vi "pll.vi"() -> ()   [LabVIEW 2020]
uses:
  <vilib>/Analysis/2dsp.llb/Real FFT.vi
  <vilib>/Analysis/baseanly.llb/Mean (DBL).vi
  <vilib>/Analysis/NI_AALBase.lvlib
  <vilib>/Analysis/NI_AALPro.lvlib
panel:
  out "Phase":dbl
  out "Input and Output Spectrum":waveform(dbl)[](graph)
  in  "milliseconds to wait":u32
  in  "iteration count":i32
  out "Input and Output vs Time":waveform(dbl)[](graph)
  in  "Loop Gain":dbl
  in  "Filter Length":i32=128
  in  "FFT size":i32=-1
  out "Frequency Estimate (Hz)":dbl
  in  "Sampling Frequency":dbl=0.0078125 format="%0.4e"
  in  "samples":i32=128
  in  "frequency":dbl=0.0078125 format="%0.4e"
  in  "phase in":dbl format="%0.2f"
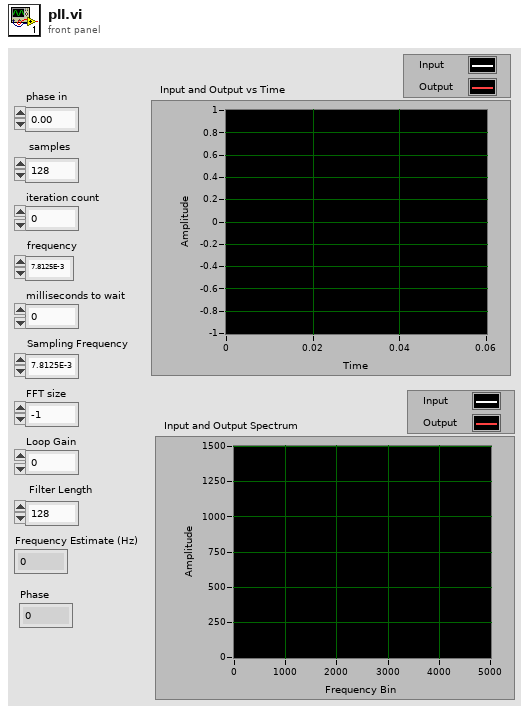
[diagram p1: front panel]
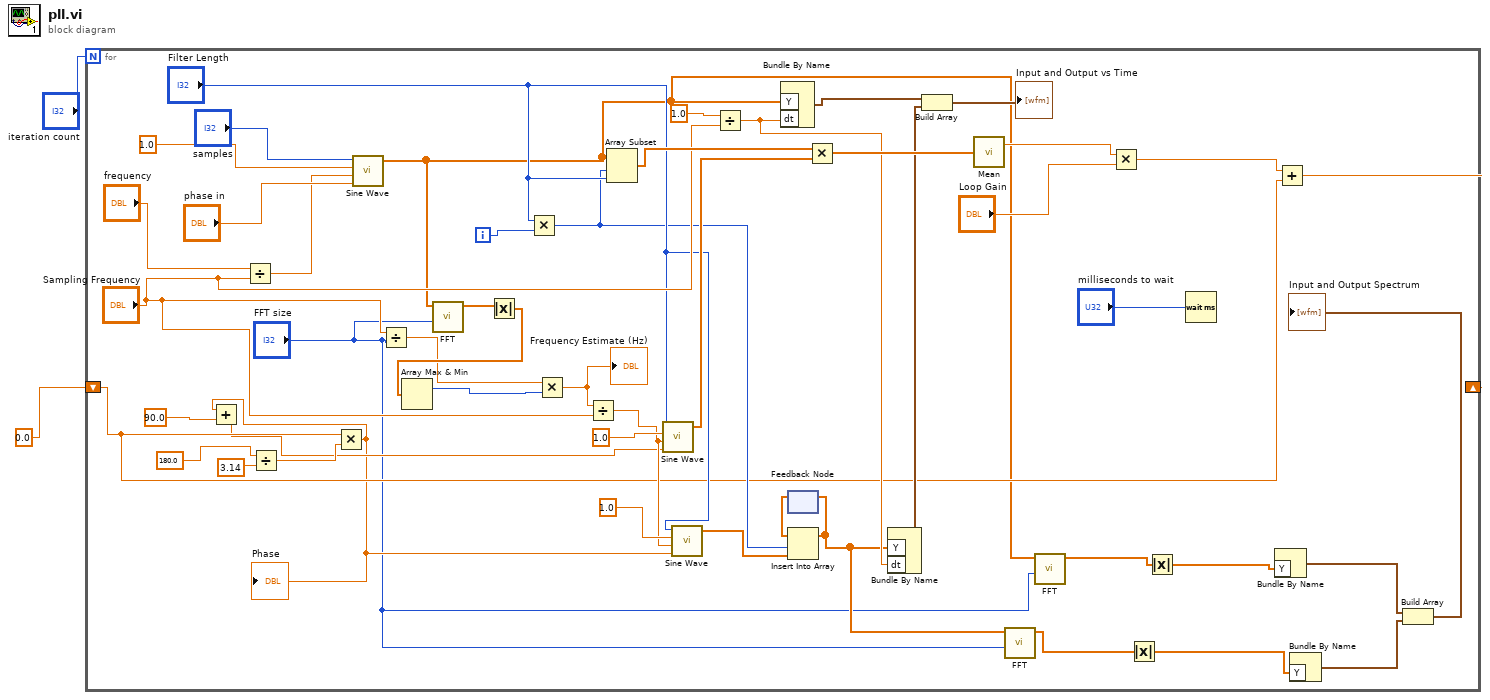
[diagram p0: block diagram]
diagram:
  n1 = for {
    N: "iteration count" -> [_]
    shift-right: [w21] -> _
    shift-left: 0.0 -> [w15]
    i -> [w33]
    n2 = Divide(x="frequency", y="Sampling Frequency") -> (x/y=w44:dbl)
    n3 = Divide(x=180.0, y=3.14) -> (x/y=w16:dbl)
    n4 = Multiply(x=w15, y=w16) -> (x*y=w13:dbl)
    "Phase" <- w13
    n5 = Add(x=w13, y=90.0) -> (x+y=w14:dbl)
    n6 = call <vilib>:"Sine Wave.vi"("samples"="samples", "amplitude"=1.0, "frequency"=w44, "phase in"="phase in") -> ("sine wave"=w10:dbl[])  [unwired: 1 in, 2 out]
    n7 = Divide(x="Sampling Frequency", y="FFT size") -> (x/y=w43:dbl)
    n8 = call-poly <vilib>:"FFT.vi"("FFT size"="FFT size", "X"=w10) -> ("FFT {X}"=w46:cdb[])  [unwired: 8 in, 1 out]
    n9 = Absolute Value(x=w46) -> (abs(x)=w45:dbl[])
    n10 = Array Max & Min(array=w45) -> (max index (indices)=w47:i32)  [unwired: 3 out]
    n11 = Multiply(x="Filter Length", y=w33) -> (x*y=w20:i32)
    n12 = Multiply(x=w43, y=w47) -> (x*y=w27:dbl)
    "Frequency Estimate (Hz)" <- w27
    n13 = Divide(x=w27, y="Sampling Frequency") -> (x/y=w25:dbl)
    n14 = Array Subset(array=w10, index=w20, length="Filter Length") -> (w39:dbl[])
    n15 = call <vilib>:"Sine Wave.vi"("samples"="Filter Length", "amplitude"=1.0, "frequency"=w25, "phase in"=w14) -> ("sine wave"=w38:dbl[])  [unwired: 1 in, 2 out]
    n16 = call <vilib>:"Sine Wave.vi"("samples"="Filter Length", "amplitude"=1.0, "frequency"=w25, "phase in"=w13) -> ("sine wave"=w31:dbl[])  [unwired: 1 in, 2 out]
    n17 = Divide(x=1.0, y="Sampling Frequency") -> (x/y=w19:dbl)
    n18 = Bundle By Name("Y"=w10, "dt"=w19) -> (w30:waveform(dbl))  [unwired: 1 in]
    n19 = feedback #1() -> (w32:dbl[])  [unwired: 1 in]
    n20 = Insert Into Array(array=w32, index=w20, new element=w31) -> (w12:dbl[])
    n21 = feedback-in #1(w12) -> ()
    n22 = Multiply(x=w39, y=w38) -> (x*y=w37:dbl[])
    n23 = Bundle By Name("Y"=w12, "dt"=w19) -> (w29:waveform(dbl))  [unwired: 1 in]
    n24 = Build Array(w30, w29) -> (→"Input and Output vs Time":waveform(dbl)[])
    n25 = call-poly <vilib>:"Mean.vi"("X"=w37) -> ("mean"=w36:dbl)  [unwired: 1 out]
    n26 = call-poly <vilib>:"FFT.vi"("FFT size"="FFT size", "X"=w12) -> ("FFT {X}"=w8:cdb[])  [unwired: 8 in, 1 out]
    n27 = call-poly <vilib>:"FFT.vi"("FFT size"="FFT size", "X"=w10) -> ("FFT {X}"=w9:cdb[])  [unwired: 8 in, 1 out]
    n28 = Multiply(x=w36, y="Loop Gain") -> (x*y=w22:dbl)
    n29 = Absolute Value(x=w8) -> (abs(x)=w7:dbl[])
    n30 = Absolute Value(x=w9) -> (abs(x)=w6:dbl[])
    n31 = Wait (ms)(milliseconds to wait="milliseconds to wait") -> ()  [unwired: 1 out]
    n32 = Bundle By Name("Y"=w6) -> (w5:waveform(dbl))  [unwired: 1 in]
    n33 = Add(x=w22, y=w15) -> (x+y=w21:dbl)
    n34 = Bundle By Name("Y"=w7) -> (w4:waveform(dbl))  [unwired: 1 in]
    n35 = Build Array(w5, w4) -> (→"Input and Output Spectrum":waveform(dbl)[])
  }
